vi "Encoder_Setup.vi"(11 "Left_Drive_Speed":T1) -> (3 "Left_Drive_Distance":dbl)   [LabVIEW 2014]
uses:
  <vilib>/Rock Robotics/WPI/Encoder/WPI_EncoderDevRef.ctl
  <vilib>/Rock Robotics/SystemInterfaces/Encoder/FPGA_EncoderIdx.ctl
  <vilib>/Rock Robotics/SystemInterfaces/Counter/FPGA_CounterCtrSystemIndex.ctl
  <vilib>/Rock Robotics/WPI/Encoder/WPI_EncoderType.ctl
  General_VI/Global Var.vi
panel:
  in  "Reset_Encoder":bool
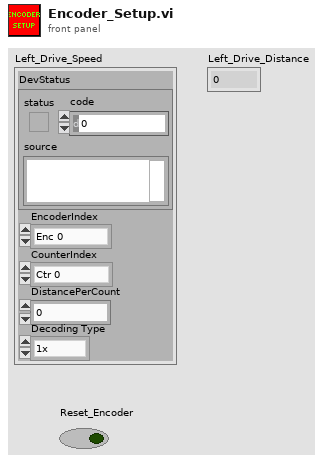
[diagram p1: front panel]
types:
  T1 = typedef "WPI_EncoderDevRef.ctl" = cluster{"DevStatus":errorcluster, "EncoderIndex":T2, "CounterIndex":T3, "DistancePerCount":dbl, "Decoding Type":T4}
  T2 = typedef "FPGA_EncoderIdx.ctl" = enum8{"Enc 0", "Enc 1", "Enc 2", "Enc 3", "Enc 4", "Enc 5", "Enc 6", "Enc 7", "Invalid"}
  T3 = typedef "FPGA_CounterCtrSystemIndex.ctl" = enum8{"Ctr 0", "Ctr 1", "Ctr 2", "Ctr 3", "Ctr 4", "Ctr 5", "Ctr 6", "Ctr 7", "Invalid"}
  T4 = typedef "WPI_EncoderType.ctl" = enum16{"1x", "2x", "4x"}
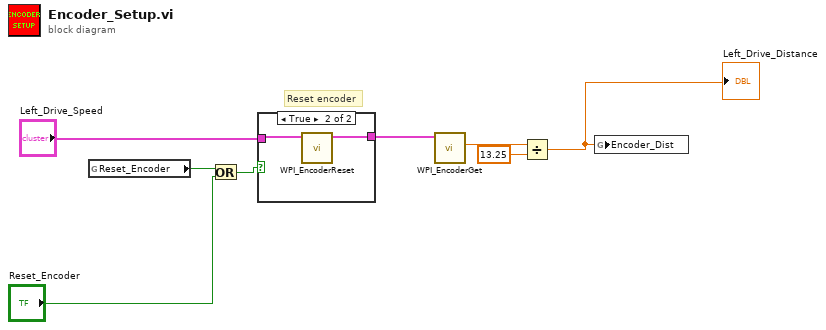
[diagram p0: block diagram]
diagram:
  # "Reset encoder"
  n1 = global read "Global Var.vi" "Reset_Encoder"() -> (w6:bool)
  n2 = Or(x=w6, y="Reset_Encoder") -> (x .or. y?=w5:bool)
  n3 = case shown="True" w5 {
    tunnel: "Left_Drive_Speed" -> [w9 w11]
    tunnel: [w9 w10] -> w8
    frame False {
    }
    frame True {
      n4 = call <vilib>:"WPI_EncoderReset.vi"("EncoderDevRef"=w11) -> ("EncoderDevRef"=w10:T1)  [unwired: 9 in, 1 out]
    }
  }
  n5 = call <vilib>:"WPI_EncoderGet.vi"("EncoderDevRef"=w8) -> ("Distance"=w3:dbl)  [unwired: 5 in, 5 out]
  n6 = Divide(x=w3, y=13.25) -> (x/y=w1:dbl)
  "Left_Drive_Distance" <- w1
  n7 = global write "Global Var.vi" "Encoder_Dist"(w1) -> ()
